vi "Read files ALL(Delay).vi"(11 "Path":path) -> (2 "Graph":dynamicdata(graph), 3 "Table":string[][](table))   [LabVIEW 2020, in "GPP.lvlib"]
uses:
  GPP.lvlib
panel:
  out "VOLTAGE":dbl[](array[numeric])
  out "TIME":dbl[](array[numeric])
  out "V":dbl
  out "T":dbl
  out "N":dbl
  out "NUMBER":dbl[](array[numeric])
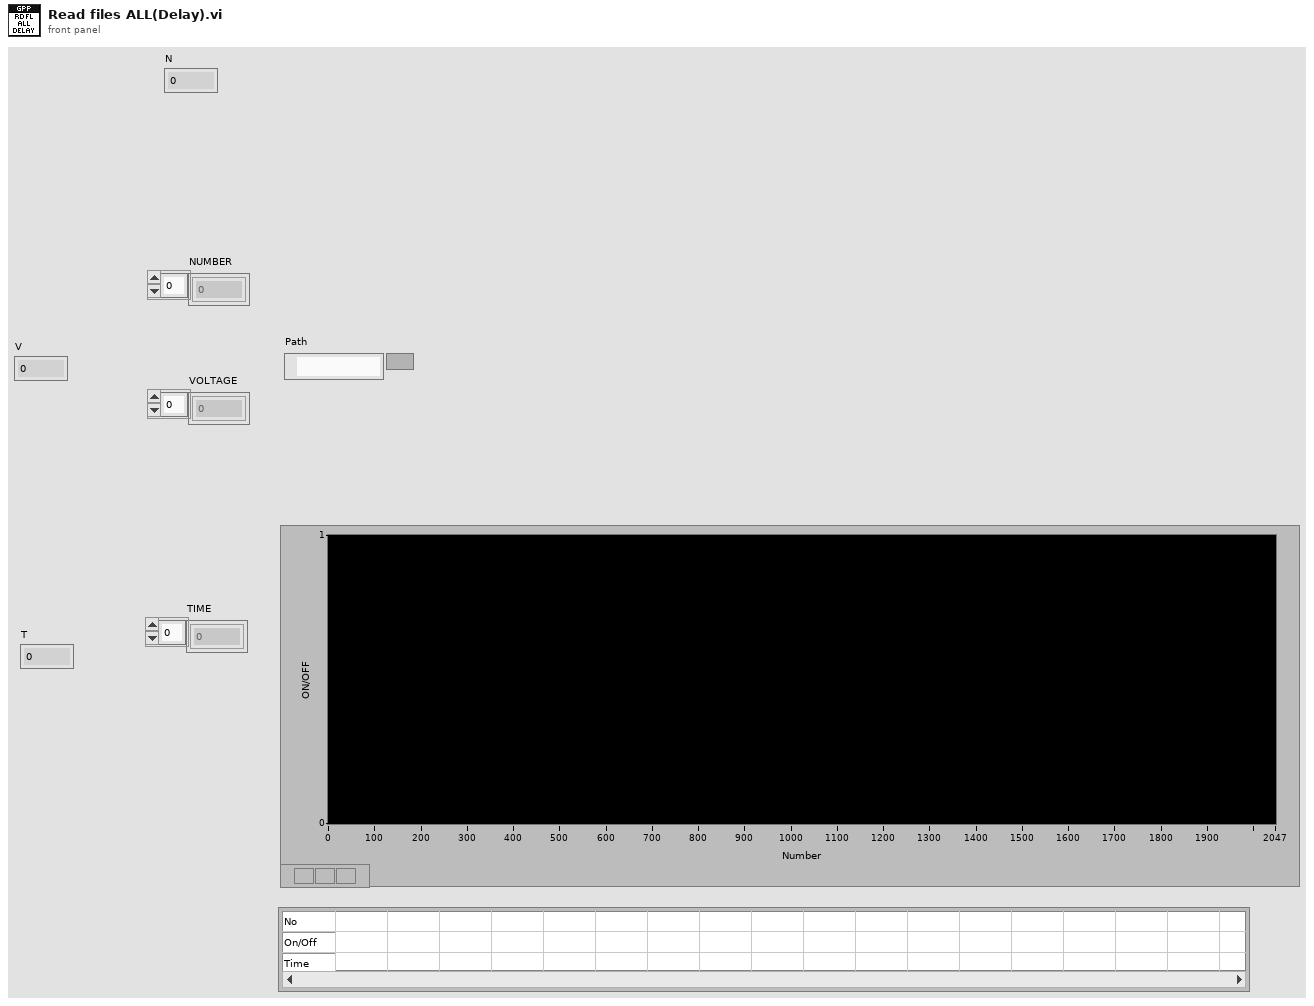
[diagram p1: front panel]
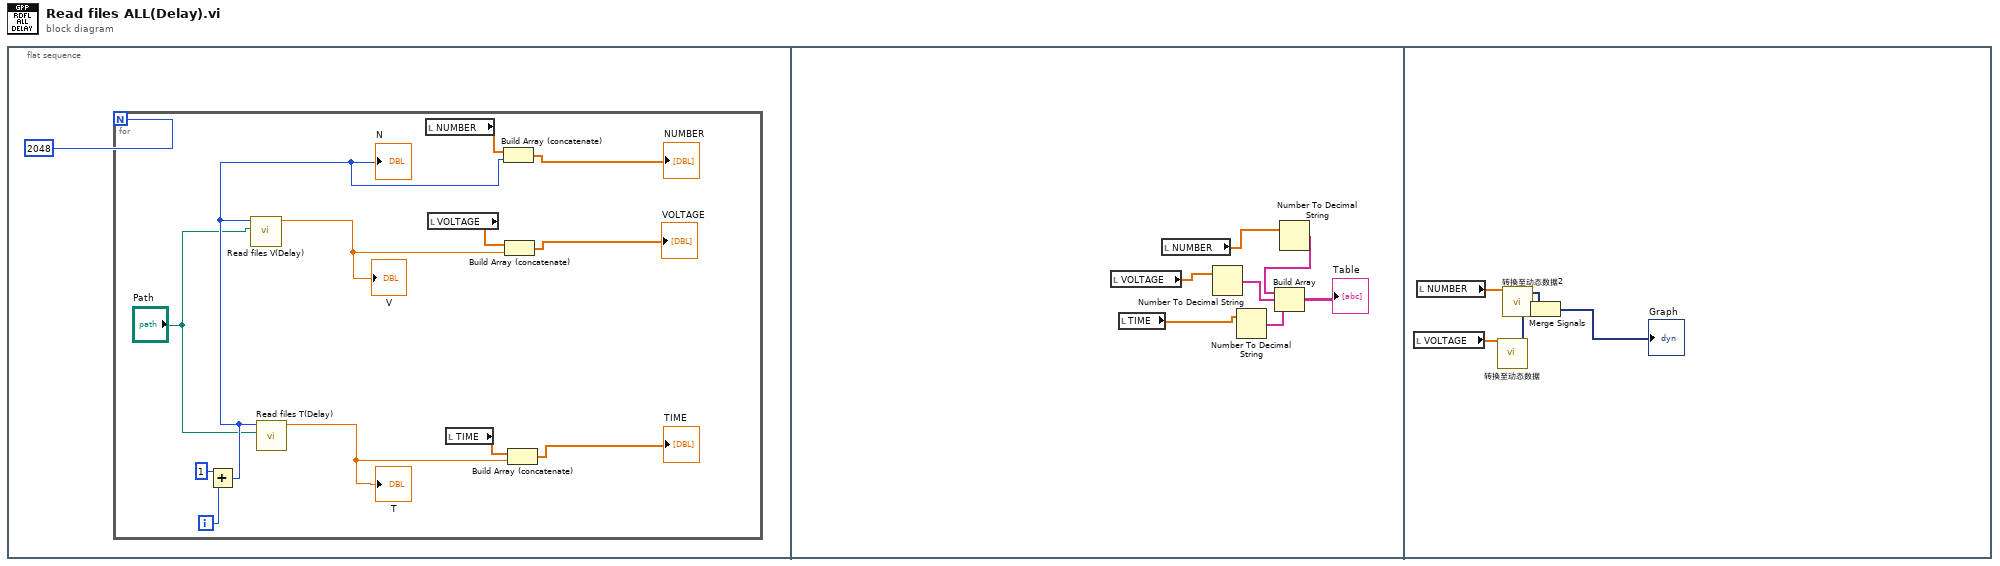
[diagram p0: block diagram]
diagram:
  n1 = flat-sequence {
    frame #0 {
      n2 = for {
        N: 2048 -> [_]
        i -> [w7]
        n3 = Add(x=1, y=w7) -> (x+y=w4:i32)
        "N" <- w4
        n4 = call "Read files V(Delay).vi"("Path"="Path", "Number"=w4) -> ("V"=w13:dbl)  [unwired: 9 in]
        "V" <- w13
        n5 = call "Read files T(Delay).vi"("Path"="Path", "Number"=w4) -> ("Time"=w12:dbl)  [unwired: 9 in]
        "T" <- w12
        n6 = local read "NUMBER"() -> (w5:dbl[])
        n7 = local read "VOLTAGE"() -> (w11:dbl[])
        n8 = local read "TIME"() -> (w10:dbl[])
        n9 = Build Array (concatenate)(w5, w4) -> (→"NUMBER":dbl[])
        n10 = Build Array (concatenate)(w11, w13) -> (→"VOLTAGE":dbl[])
        n11 = Build Array (concatenate)(w10, w12) -> (→"TIME":dbl[])
      }
    }
    frame #1 {
      n12 = local read "VOLTAGE"() -> (w15:dbl[])
      n13 = local read "TIME"() -> (w20:dbl[])
      n14 = local read "NUMBER"() -> (w16:dbl[])
      n15 = Number To Decimal String(number=w15) -> (decimal integer string=w14:string[])  [unwired: 1 in]
      n16 = Number To Decimal String(number=w20) -> (decimal integer string=w19:string[])  [unwired: 1 in]
      n17 = Number To Decimal String(number=w16) -> (decimal integer string=w18:string[])  [unwired: 1 in]
      n18 = Build Array(w18, w14, w19) -> (→"Table":string[][])
    }
    frame #2 {
      n19 = local read "VOLTAGE"() -> (w25:dbl[])
      n20 = local read "NUMBER"() -> (w21:dbl[])
      n21 = call "转换至动态数据"("Array"=w25) -> ("Dynamic Data Type"=w22:dynamicdata)  [unwired: 3 in]
      n22 = call "转换至动态数据2"("Array"=w21) -> ("Dynamic Data Type"=w24:dynamicdata)  [unwired: 3 in]
      n23 = Merge Signals(w24, w22) -> (→"Graph":dynamicdata)
    }
  }
